vi "circular_calc_desired_position.vi"(0 "Current Position":dbl, 1 "Reset":bool=TRUE, 5 "Driver Input":dbl, 7 "Max Velocity":dbl, 9 "Scale Factor":dbl, 11 "dt":dbl, 12 "Upper Bound":dbl, 13 "Lower Bound":dbl) -> (4 "Desired Position":dbl)   [LabVIEW 2012]
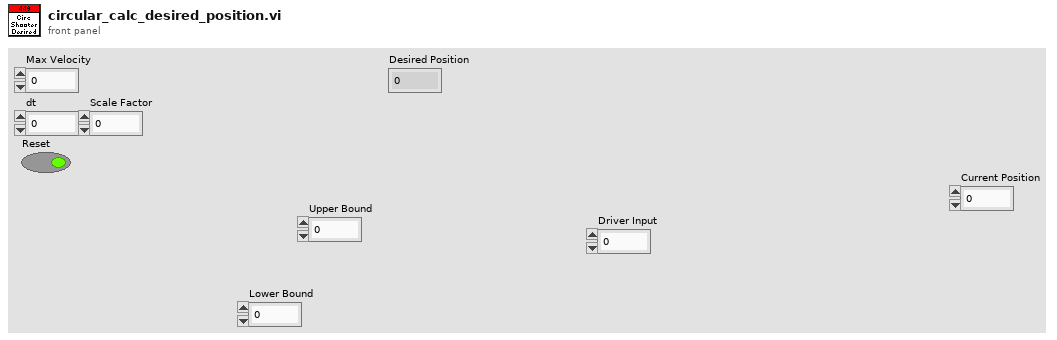
[diagram p1: front panel]
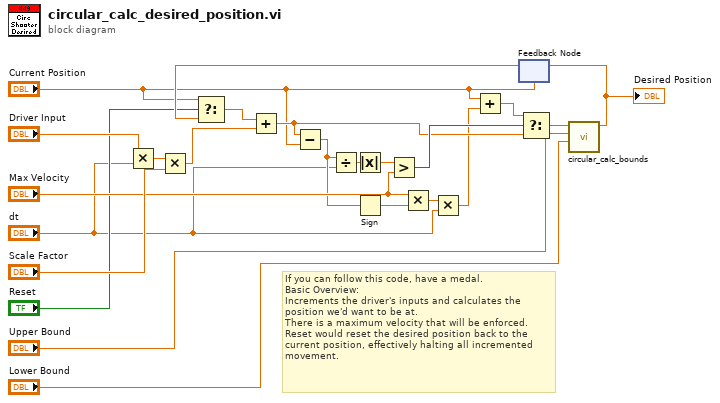
[diagram p0: block diagram]
diagram:
  # "If you can follow this code, have a medal.\nBasic Overview:\nIncrements the driver's inputs and calculates the\nposition we'd want to be at.\nThere is a maximum velocity that will be enforced.\nReset would reset the desired position back to the\ncurrent position, effectively halting all incremented\nmovement."
  n1 = Multiply(x="Driver Input", y="dt") -> (x*y=w19:dbl)
  n2 = Multiply(x=w19, y="Scale Factor") -> (x*y=w22:dbl)
  n3 = feedback #1("Current Position") -> (w23:dbl)
  n4 = Select(t="Current Position", s="Reset", f=w23) -> (s? t:f=w12:dbl)
  n5 = Add(x=w12, y=w22) -> (x+y=w16:dbl)
  n6 = Subtract(x=w16, y="Current Position") -> (x-y=w10:dbl)
  n7 = Divide(x=w10, y="dt") -> (x/y=w7:dbl)
  n8 = Absolute Value(x=w7) -> (abs(x)=w18:dbl)
  n9 = Sign(1:w10) -> (0:w14:dbl)
  n10 = Greater?(x=w18, y="Max Velocity") -> (0:w17:bool)
  n11 = Multiply(x="Max Velocity", y=w14) -> (x*y=w13:dbl)
  n12 = Multiply(x=w13, y="dt") -> (x*y=w6:dbl)
  n13 = Add(x="Current Position", y=w6) -> (x+y=w9:dbl)
  n14 = Select(t=w9, s=w17, f=w16) -> (s? t:f=w2:dbl)
  n15 = call "circular_calc_bounds.vi"("Lower Bound"="Lower Bound", "Upper Bound"="Upper Bound", "Desired Position"=w2) -> ("Desired Position Out"=w1:dbl)  [unwired: 8 in]
  "Desired Position" <- w1
  n16 = feedback-in #1(w1) -> ()
